vi "File tab event details.vi"(0 "stop":bool, 5 "Ring 2":u16(ring) items=["Event 2.txt", "License Key (1).txt", "License Key.txt", "Pinnacle 19.5 + Efeitos.txt"], 8 "y":bool, 11 "Select Folder":bool) -> (2 "Event Details :":string)   [LabVIEW 2014]
panel:
  out "Path 3":path
  out "Path 2":path
  out "result string":string
  out "element 2":bool
  out "element":string
  out "Numeric":dbl
  out "filenames 2":string[](array[string])
  out "filenames":string[](array[string])
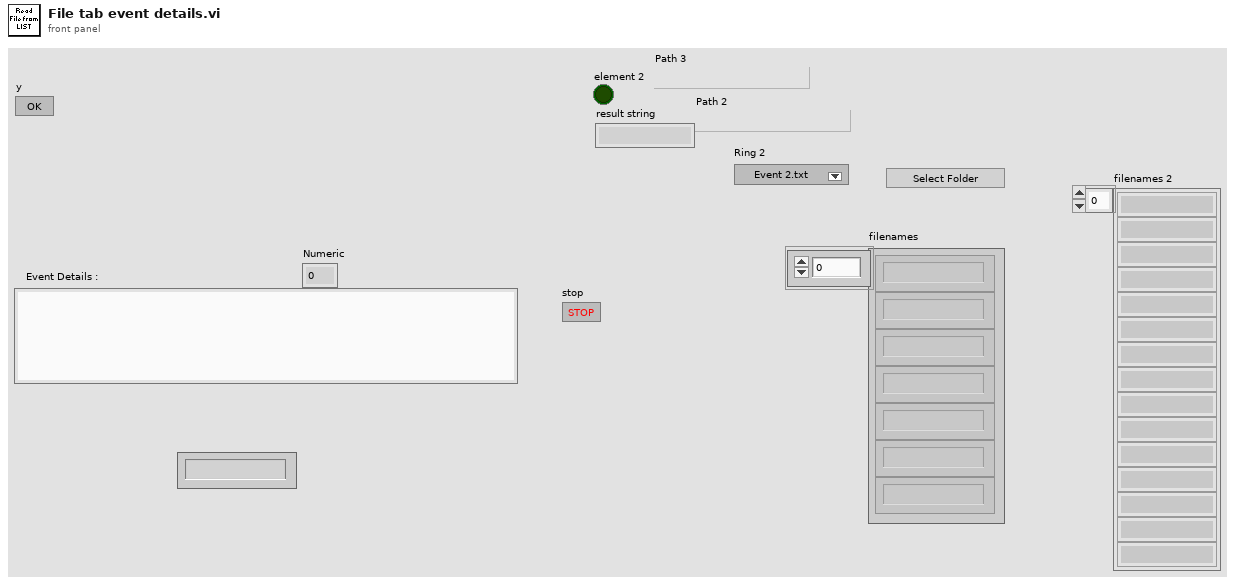
[diagram p1: front panel]
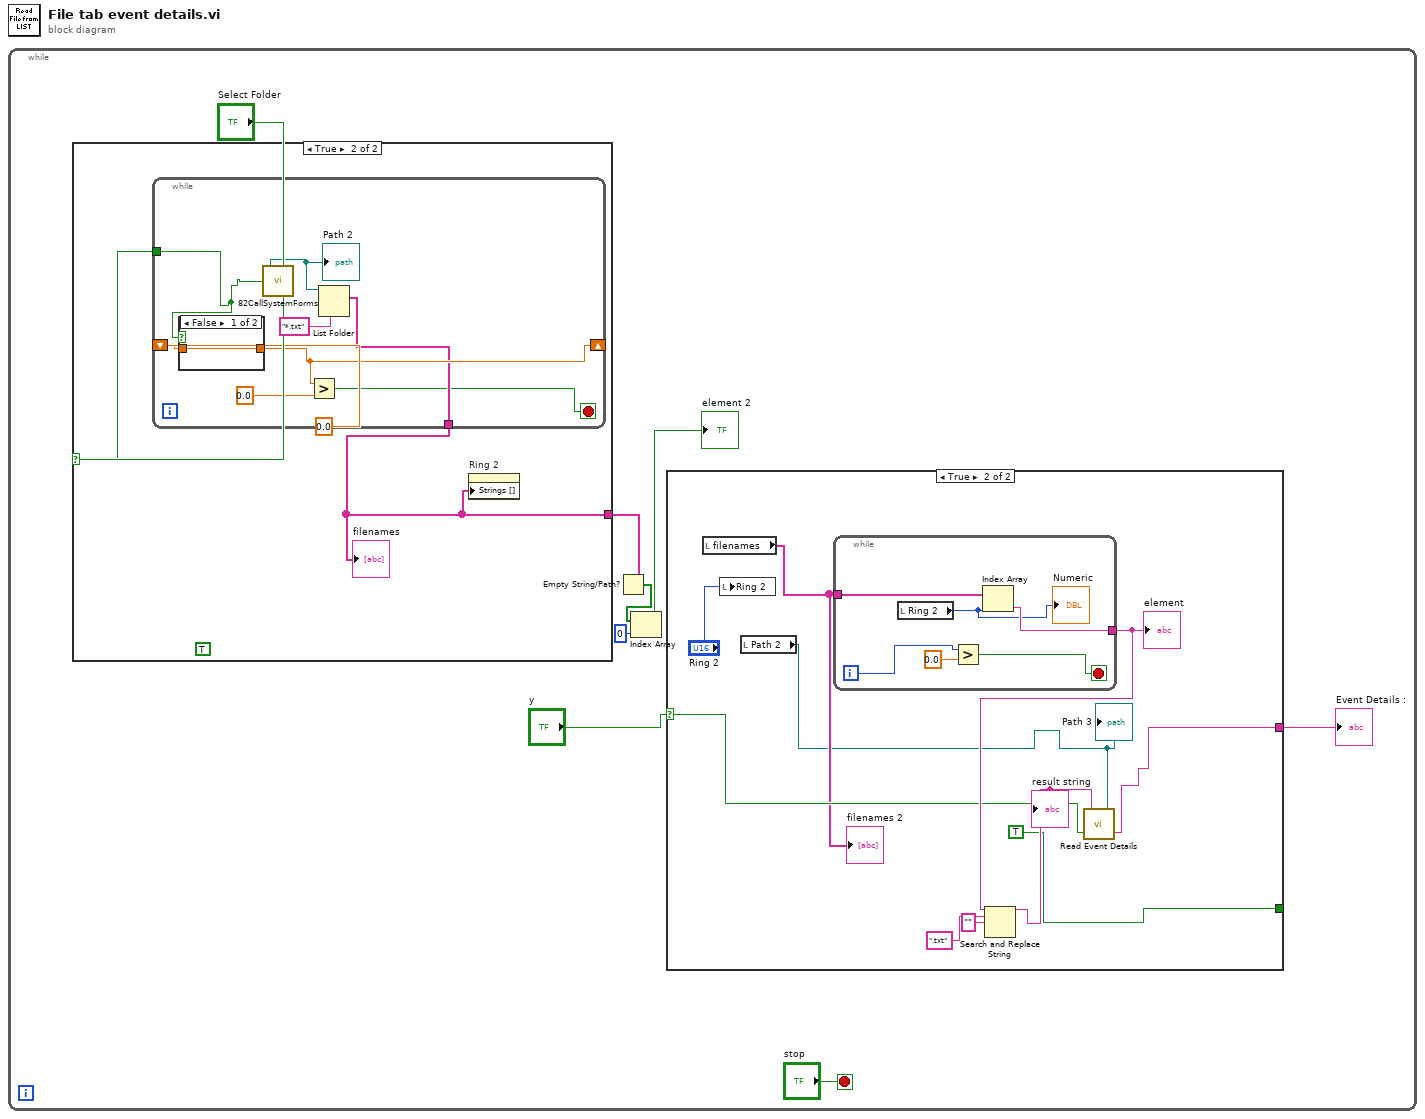
[diagram p0: block diagram]
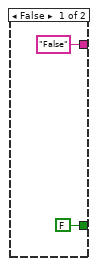
[diagram p2: hidden frame]
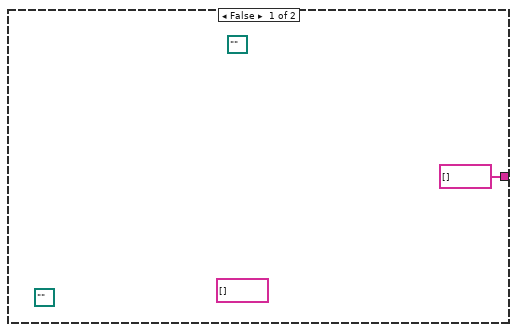
[diagram p3: hidden frame]
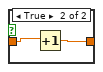
[diagram p4: hidden frame]
diagram:
  n1 = while {
    stop <- "stop" stop-if-true
    n2 = case shown="True" "Select Folder" {
      selector: "Select Folder" -> [_ w29]
      tunnel: [string[] [] ("filenames") w28] -> w6
      frame False {
        (unwired) path "" ("Path")
        (unwired) path "" ("Path")
        (unwired) string[] [] ("filenames")
      }
      frame True {
        (unwired) TRUE
        n3 = while {
          shift-right: [w35] -> _
          shift-left: 0.0 ("Numeric") -> [w36]
          tunnel: [w34] -> w28
          tunnel: w29 -> [w32]
          stop <- w33 stop-if-true
          n4 = case shown="False" w32 {
            tunnel: w36 -> [w39 w41]
            tunnel: [w39 w40] -> w35
            frame False {
            }
            frame True {
              n5 = Increment(x=w41) -> (x+1=w40:dbl)
            }
          }
          n6 = call "82CallSystemForms.vi"("OK Button"=w32) -> ("Path"=w31:path)  [unwired: 1 in, 2 out]
          "Path 2" <- w31
          n7 = Greater?(x=w35, y=0.0 ("Numeric")) -> (0:w33:bool)
          n8 = List Folder(path=w31, pattern="*.txt") -> (filenames=w34:string[])  [unwired: 2 in, 3 out]
        }
        "filenames" <- w28
        n9 = property on="Ring 2" class="Ring (strict)"("Strings []"=w28) -> ()  [unwired: 2 in, 2 out]
      }
    }
    n10 = Empty String/Path?(string/path=w6) -> (empty?=w5:bool[])
    n11 = Index Array(array=w5, index=0) -> (element=→"element 2":bool)
    n12 = case shown="True" "y" {
      selector: "y" -> [_ w16]
      tunnel: [FALSE ("Boolean") TRUE ("Boolean")] -> _
      tunnel: ["False" ("text") w12] -> w1
      frame False {
      }
      frame True {
        n13 = local read "filenames"() -> (w15:string[])
        "filenames 2" <- w15
        n14 = local write "Ring 2"("Ring 2") -> ()
        n15 = local read "Path 2"() -> (w11:path)
        "Path 3" <- w11
        n16 = while {
          tunnel: [w26] -> w17
          tunnel: w15 -> [w21]
          i -> [w23]
          stop <- w24 stop-if-true
          n17 = local read "Ring 2"() -> (w22:u16)
          "Numeric" <- w22
          n18 = Greater?(x=w23, y=0.0) -> (0:w24:bool)
          n19 = Index Array(array=w21, index=w22) -> (element=w26:string)
        }
        "element" <- w17
        n20 = Search and Replace String(input string=w17, search string=".txt" ("substring (\"\")"), replace string="" ("replace string (\"\")")) -> (result string=w18:string)  [unwired: 5 in, 3 out]
        "result string" <- w18
        n21 = call "Read Event Details.vi"("path"=w11, "OK Button"=w16, "Event Name"=w18) -> ("text"=w12:string)
      }
    }
    "Event Details :" <- w1
  }
